vi "ReadALetter.vi"(10 "all rows 3":dbl[][](array[numeric]), 11 "x":dbl) -> (2 "Array 3":dbl[](array[numeric]), 3 "Array 4":dbl[](array[numeric]))   [LabVIEW 2018]
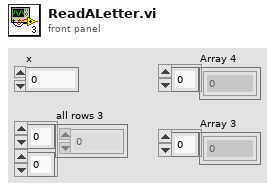
[diagram p1: front panel]
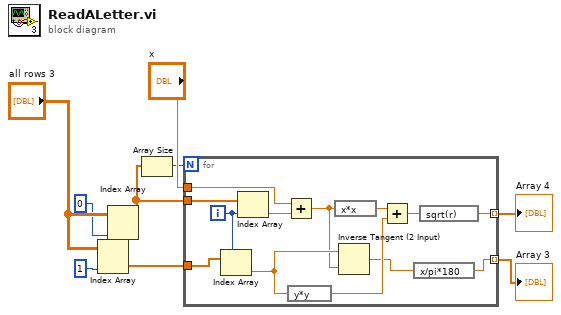
[diagram p0: block diagram]
diagram:
  n1 = Index Array(array="all rows 3", index (col)=1 ("disabled index (col)")) -> (element=w3:dbl[])  [unwired: 1 in]
  n2 = Index Array(array="all rows 3", index (col)=0 ("disabled index (col)")) -> (element=w4:dbl[])  [unwired: 1 in]
  n3 = Array Size(array=w4) -> (size(s)=w6:i32)
  n4 = for {
    N: w6 -> [_]
    tunnel: w4 -> [w22]
    tunnel: w3 -> [w18]
    tunnel: [w14] -> w2 mode=indexing
    tunnel: [w13] -> w1 mode=indexing
    tunnel: "x" -> [w10]
    i -> [w19]
    n5 = Index Array(array=w18, index=w19) -> (element=w15:dbl)
    n6 = Index Array(array=w22, index=w19) -> (element=w12:dbl)
    n7 = Add(x=w10, y=w12) -> (x+y=w11:dbl)
    n8 = expression code="y*y"(w15) -> (w17:dbl)
    n9 = expression code="x*x"(w11) -> (w20:dbl)
    n10 = Inverse Tangent (2 Input)(1:w11, 2:w15) -> (0:w16:dbl)
    n11 = Add(x=w20, y=w17) -> (x+y=w21:dbl)
    n12 = expression code="x/pi*180"(w16) -> (w14:dbl)
    n13 = expression code="sqrt(r)"(w21) -> (w13:dbl)
  }
  "Array 3" <- w2
  "Array 4" <- w1
